vi "datasource.to_json.vi"(8 "error in":errorcluster, 10 "dataSource":T1) -> (0 "error out":errorcluster, 2 "json":string)   [LabVIEW 2020, in "dataScopes.lvlib"]
uses:
  dataScopes.lvlib
  <vilib>/JDP Science/JSONtext/JSONtext.lvlib
  ab7c0d24-36bc-4d84-84a5-6341875158a7.vi
  505a04b1-beae-45fc-bcd5-c0218de0aff1.vi
  type.ctl
  data_source.ctl
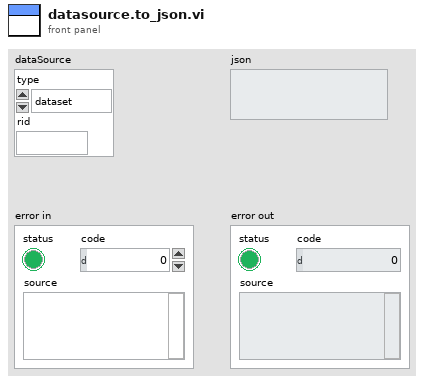
[diagram p1: front panel]
types:
  T1 = typedef "dataScopes.lvlib/data_source.ctl" = cluster{"type":T2, "rid":string}
  T2 = typedef "dataScopes.lvlib/type.ctl" = enum16{"dataset", "connection", "logSet", "video"}
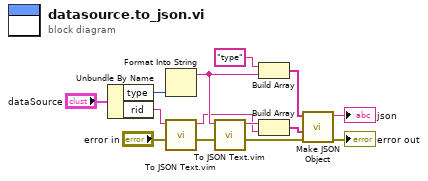
[diagram p0: block diagram]
diagram:
  n1 = Unbundle By Name("dataSource") -> ("type"=w13:T2, "rid"=w10:string)
  n2 = Format Into String(w13) -> (resulting string=w9:string)  [unwired: 3 in, 1 out]
  n3 = call "To JSON Text.vim"("error in (no error)"="error in", "Anything"=w10) -> ("error out"=w4:errorcluster, "<JSON>"=w7:string)  [unwired: 8 in]
  n4 = call "To JSON Text.vim"("error in (no error)"=w4, "Anything"=w9) -> ("error out"=w3:errorcluster, "<JSON>"=w8:string)  [unwired: 8 in]
  n5 = Build Array("type", w9) -> (w11:string[])
  n6 = Build Array(w8, w7) -> (w6:string[])
  n7 = call <vilib>:"Make JSON Object.vi"("error in (no error)"=w3, "JSON Items"=w6, "Item Names"=w11) -> ("error out"=→"error out":errorcluster, "<JSON>"=→"json":string)  [unwired: 7 in]
